vi "Write Controls to Config File.vi"(6 "Child?":bool, 7 "section":string, 8 "Error In":errorcluster, 9 "ParentName":string, 10 "Ctl Refnum":refnum<vi>, 11 "refnum":T1) -> (0 "Error Out":errorcluster, 3 "refnum out":T1)   [LabVIEW 2017]
uses:
  <vilib>/Utility/config.llb/Config Data RefNum.ctl
  Hardware/Table Stage/Controls/Translation Stage Cluster.ctl
  Controls/Translation Stage Types.ctl
  <vilib>/Utility/config.llb/Write Key (String).vi
  <vilib>/Utility/config.llb/Write Key (Path).vi
  <vilib>/Utility/config.llb/Write Key (Boolean).vi
  <vilib>/Utility/config.llb/Write Key (Double).vi
  <vilib>/Utility/config.llb/Write Key (U32).vi
  <vilib>/Utility/config.llb/NI_LVConfig.lvlib
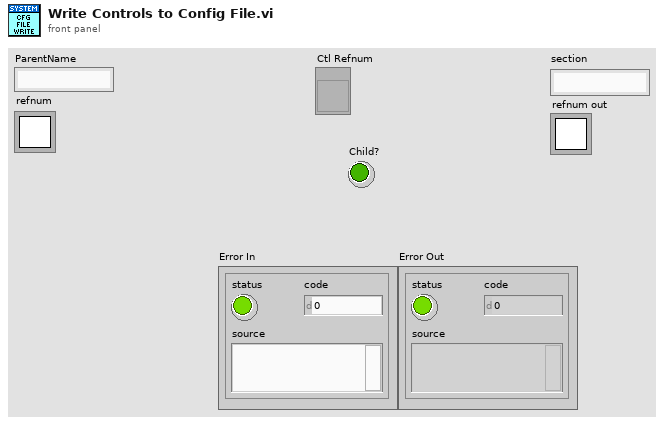
[diagram p1: front panel]
types:
  T1 = typedef "NI_LVConfig.lvlib/Config Data RefNum.ctl" = refnum<k1>
  T2 = typedef "Translation Stage Cluster.ctl" = cluster{"Position":dbl, "Is.Enabled?":bool, "Is.Connected?":bool, "Device SN":string, "AccelerationMaximum":dbl, "VelocityMaximum":dbl, "Acceleration":dbl, "Velocity":dbl, "waitTimeout (ms)":i32, "Model":T3, "Is.Homed?":bool}
  T3 = typedef "Translation Stage Types.ctl" = enum16{"None", "Thorlabs LTS", "Thorlabs MLJ"}
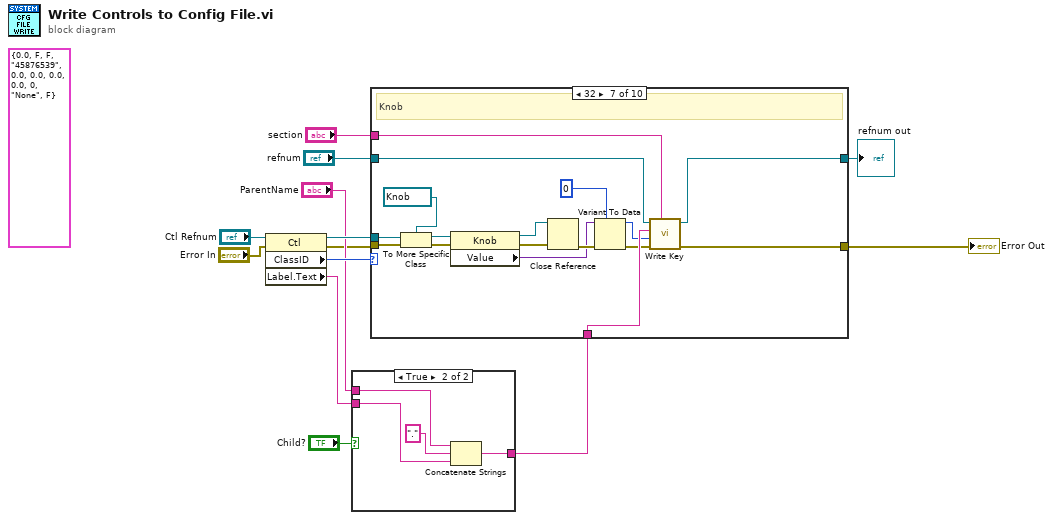
[diagram p0: block diagram]
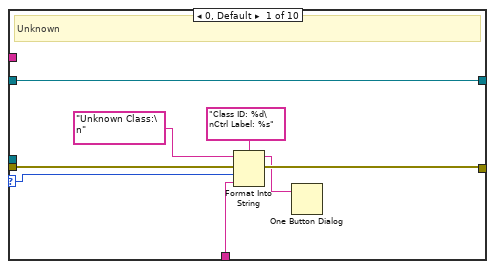
[diagram p3: hidden frame]
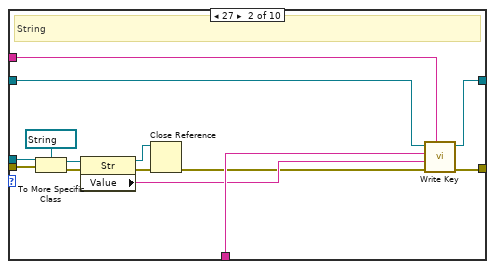
[diagram p4: hidden frame]
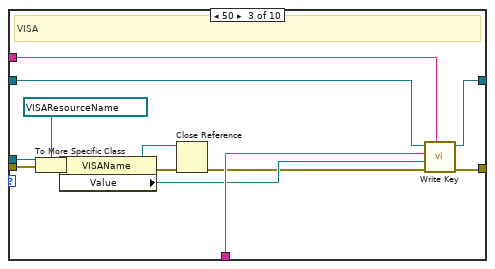
[diagram p5: hidden frame]
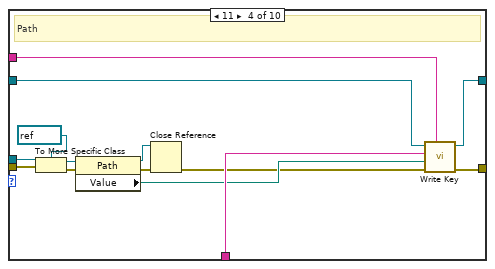
[diagram p6: hidden frame]
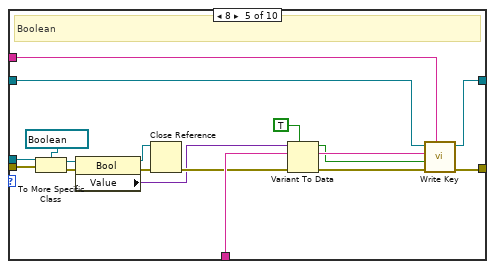
[diagram p7: hidden frame]
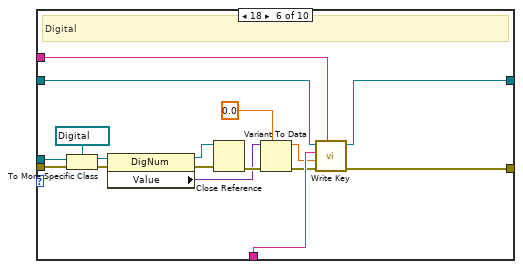
[diagram p8: hidden frame]
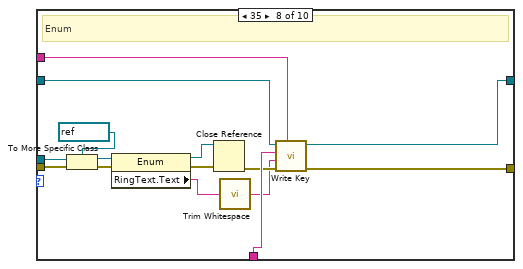
[diagram p9: hidden frame]
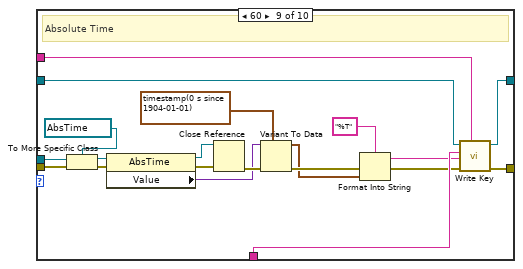
[diagram p10: hidden frame]
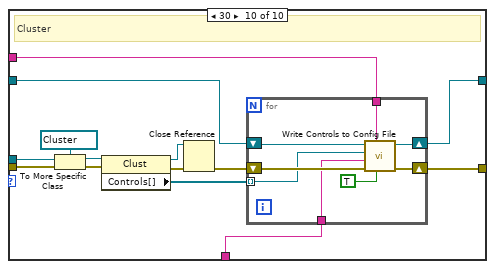
[diagram p11: hidden frame]
diagram:
  (unwired) T2 {"Position"=0.0, "Is.Enabled?"=FALSE, "Is.Connected?"=FALSE, "Device SN"="45876539", "AccelerationMaximum"=0.0, "VelocityMaximum"=0.0, "Acceleration"=0.0, "Velocity"=0.0, "waitTimeout (ms)"=0, "Model"=enum."None", "Is.Homed?"=FALSE} ("Control Param In")
  n1 = property class="Ctl"(reference="Ctl Refnum", error in="Error In") -> (reference out=w12:refnum<vi>, error out=w6:errorcluster, "ClassID"=w11:u32, "Label.Text"=w8:string)
  n2 = case shown="True" "Child?" {
    tunnel: "ParentName" -> [_ w18]
    tunnel: w8 -> [w14 w16]
    tunnel: [w14 w15] -> w3
    frame False {
    }
    frame True {
      n3 = Concatenate Strings(w18, ".", w16) -> (w15:string)
    }
  }
  n4 = case shown="32" w11 {
    selector: w11 -> [w23 _ _ _ _ _ _ _ _ _]
    tunnel: w6 -> [w21 w39 w54 w68 w84 w102 w119 w134 w154 w168]
    tunnel: w12 -> [_ w38 w53 w67 w83 w101 w118 w133 w153 w166]
    tunnel: [w20 w37 w52 w66 w82 w90 w108 w124 w143 w162] -> w1
    tunnel: "section" -> [_ w36 w51 w65 w81 w93 w111 w127 w146 w159]
    tunnel: "refnum" -> [w26 w35 w50 w64 w80 w92 w110 w126 w145 w161]
    tunnel: [w26 w34 w49 w63 w79 w91 w109 w125 w144 w160] -> w2
    tunnel: w3 -> [w22 w32 w47 w61 w77 w94 w112 w128 w147 w158]
    frame 0, Default {
      # "Unknown"
      n5 = Format Into String(format string="Class ID: %d\nCtrl Label: %s", initial string="Unknown Class:\n" ("string"), error in=w21, w23, w22) -> (resulting string=w19:string, error out=w20:errorcluster)
      n6 = One Button Dialog(message=w19) -> ()  [unwired: 1 in, 1 out]
    }
    frame 27 {
      # "String"
      n7 = To More Specific Class(target class=refnum<vi> refnum ("AccelerationMaximum 2"), reference=w38, error in=w39) -> (specific class reference=w30:refnum<vi>, error out=w33:errorcluster)
      n8 = property class="Str"(reference=w30, error in=w33) -> (reference out=w27:refnum<vi>, error out=w31:errorcluster, "Value"=w29:string)
      n9 = Close Reference(reference=w27, error in (no error)=w31) -> (error out=w28:errorcluster)
      n10 = call-poly <vilib>:"Write Key.vi"("section"=w36, "error in (no error)"=w28, "value"=w29, "key"=w32, "refnum"=w35) -> ("error out"=w37:errorcluster, "refnum out"=w34:T1)  [unwired: 4 in, 1 out]
    }
    frame 50 {
      # "VISA"
      n11 = To More Specific Class(target class=refnum<vi> refnum ("Controller VISA Ref"), reference=w53, error in=w54) -> (specific class reference=w45:refnum<vi>, error out=w48:errorcluster)
      n12 = property class="VISAName"(reference=w45, error in=w48) -> (reference out=w42:refnum<vi>, error out=w46:errorcluster, "Value"=w44:refnum<visa-resource-name>)
      n13 = Close Reference(reference=w42, error in (no error)=w46) -> (error out=w43:errorcluster)
      n14 = call-poly <vilib>:"Write Key.vi"("section"=w51, "error in (no error)"=w43, "value"=w44, "key"=w47, "refnum"=w50) -> ("error out"=w52:errorcluster, "refnum out"=w49:T1)  [unwired: 4 in, 1 out]
    }
    frame 11 {
      # "Path"
      n15 = To More Specific Class(target class=refnum<vi> refnum ("Path"), reference=w67, error in=w68) -> (specific class reference=w59:refnum<vi>, error out=w62:errorcluster)
      n16 = property class="Path"(reference=w59, error in=w62) -> (reference out=w56:refnum<vi>, error out=w60:errorcluster, "Value"=w58:path)
      n17 = Close Reference(reference=w56, error in (no error)=w60) -> (error out=w57:errorcluster)
      n18 = call-poly <vilib>:"Write Key.vi"("section"=w65, "error in (no error)"=w57, "value"=w58, "key"=w61, "refnum"=w64) -> ("error out"=w66:errorcluster, "refnum out"=w63:T1)  [unwired: 4 in, 1 out]
    }
    frame 8 {
      # "Boolean"
      n19 = To More Specific Class(target class=refnum<vi> refnum ("AccelerationMaximum 2"), reference=w83, error in=w84) -> (specific class reference=w75:refnum<vi>, error out=w78:errorcluster)
      n20 = property class="Bool"(reference=w75, error in=w78) -> (reference out=w73:refnum<vi>, error out=w76:errorcluster, "Value"=w71:variant)
      n21 = Close Reference(reference=w73, error in (no error)=w76) -> (error out=w74:errorcluster)
      n22 = Variant To Data(error in=w74, type=TRUE, Variant=w71) -> (data=w69:bool, error out=w72:errorcluster)
      n23 = call-poly <vilib>:"Write Key.vi"("section"=w81, "error in (no error)"=w72, "value"=w69, "key"=w77, "refnum"=w80) -> ("error out"=w82:errorcluster, "refnum out"=w79:T1)  [unwired: 4 in, 1 out]
    }
    frame 18 {
      # "Digital"
      n24 = To More Specific Class(target class=refnum<vi> refnum ("AccelerationMaximum 2"), reference=w101, error in=w102) -> (specific class reference=w98:refnum<vi>, error out=w99:errorcluster)
      n25 = property class="DigNum"(reference=w98, error in=w99) -> (reference out=w96:refnum<vi>, error out=w97:errorcluster, "Value"=w88:variant)
      n26 = Close Reference(reference=w96, error in (no error)=w97) -> (error out=w95:errorcluster)
      n27 = Variant To Data(error in=w95, type=0.0, Variant=w88) -> (data=w86:dbl, error out=w89:errorcluster)
      n28 = call-poly <vilib>:"Write Key.vi"("section"=w93, "error in (no error)"=w89, "value"=w86, "key"=w94, "refnum"=w92) -> ("error out"=w90:errorcluster, "refnum out"=w91:T1)  [unwired: 4 in, 1 out]
    }
    frame 32 {
      # "Knob"
      n29 = To More Specific Class(target class=refnum<vi> refnum ("Zoom Factor"), reference=w118, error in=w119) -> (specific class reference=w116:refnum<vi>, error out=w117:errorcluster)
      n30 = property class="Knob"(reference=w116, error in=w117) -> (reference out=w114:refnum<vi>, error out=w115:errorcluster, "Value"=w106:variant)
      n31 = Close Reference(reference=w114, error in (no error)=w115) -> (error out=w113:errorcluster)
      n32 = Variant To Data(error in=w113, type=u32 0, Variant=w106) -> (data=w104:u32, error out=w107:errorcluster)
      n33 = call-poly <vilib>:"Write Key.vi"("section"=w111, "error in (no error)"=w107, "value"=w104, "key"=w112, "refnum"=w110) -> ("error out"=w108:errorcluster, "refnum out"=w109:T1)  [unwired: 4 in, 1 out]
    }
    frame 35 {
      # "Enum"
      n34 = To More Specific Class(target class=refnum<vi> refnum ("Enum"), reference=w133, error in=w134) -> (specific class reference=w131:refnum<vi>, error out=w132:errorcluster)
      n35 = property class="Enum"(reference=w131, error in=w132) -> (reference out=w129:refnum<vi>, error out=w130:errorcluster, "RingText.Text"=w121:string)
      n36 = Close Reference(reference=w129, error in (no error)=w130) -> (error out=w122:errorcluster)
      n37 = call <vilib>:"Trim Whitespace.vi"("string"=w121) -> ("trimmed string"=w120:string)  [unwired: 1 in]
      n38 = call-poly <vilib>:"Write Key.vi"("section"=w127, "error in (no error)"=w122, "value"=w120, "key"=w128, "refnum"=w126) -> ("error out"=w124:errorcluster, "refnum out"=w125:T1)  [unwired: 4 in, 1 out]
    }
    frame 60 {
      # "Absolute Time"
      n39 = To More Specific Class(target class=refnum<vi> refnum ("AccelerationMaximum 2"), reference=w153, error in=w154) -> (specific class reference=w151:refnum<vi>, error out=w152:errorcluster)
      n40 = property class="AbsTime"(reference=w151, error in=w152) -> (reference out=w149:refnum<vi>, error out=w150:errorcluster, "Value"=w141:variant)
      n41 = Close Reference(reference=w149, error in (no error)=w150) -> (error out=w148:errorcluster)
      n42 = Variant To Data(error in=w148, type=timestamp(0 s since 1904-01-01), Variant=w141) -> (data=w135:timestamp, error out=w142:errorcluster)
      n43 = Format Into String(format string="%T", error in=w142, w135) -> (resulting string=w139:string, error out=w140:errorcluster)  [unwired: 1 in]
      n44 = call-poly <vilib>:"Write Key.vi"("section"=w146, "error in (no error)"=w140, "value"=w139, "key"=w147, "refnum"=w145) -> ("error out"=w143:errorcluster, "refnum out"=w144:T1)  [unwired: 4 in, 1 out]
    }
    frame 30 {
      # "Cluster"
      n45 = To More Specific Class(target class=refnum<vi> refnum ("Cluster Ref In"), reference=w166, error in=w168) -> (specific class reference=w164:refnum<vi>, error out=w165:errorcluster)
      n46 = property class="Clust"(reference=w164, error in=w165) -> (reference out=w156:refnum<vi>, error out=w163:errorcluster, "Controls[]"=w155:refnum<vi>[])
      n47 = Close Reference(reference=w156, error in (no error)=w163) -> (error out=w157:errorcluster)
      n48 = for {
        tunnel: w159 -> [w172]
        tunnel: w158 -> [w171]
        shift-right: [w175] -> w162
        shift-left: w157 -> [w176]
        shift-right: [w173] -> w160
        shift-left: w161 -> [w174]
        tunnel: w155 -> [w169] mode=indexing
        n49 = call "Write Controls to Config File.vi"("Child?"=TRUE, "section"=w172, "Error In"=w176, "ParentName"=w171, "Ctl Refnum"=w169, "refnum"=w174) -> ("Error Out"=w175:errorcluster, "refnum out"=w173:T1)  [unwired: 4 in]
      }
    }
  }
  "Error Out" <- w1
  "refnum out" <- w2
